vi "manage errors.vi"(8 "error in (no error)":errorcluster, 11 "Channel in":refnum<class "Channel.lvclass">) -> (0 "error out":errorcluster, 1 "sys error":errorcluster, 2 "exe error":errorcluster, 3 "Channel out":refnum<class "Channel.lvclass">)   [LabVIEW 2018, in "Channel.lvclass"]
uses:
  Channel.lvclass
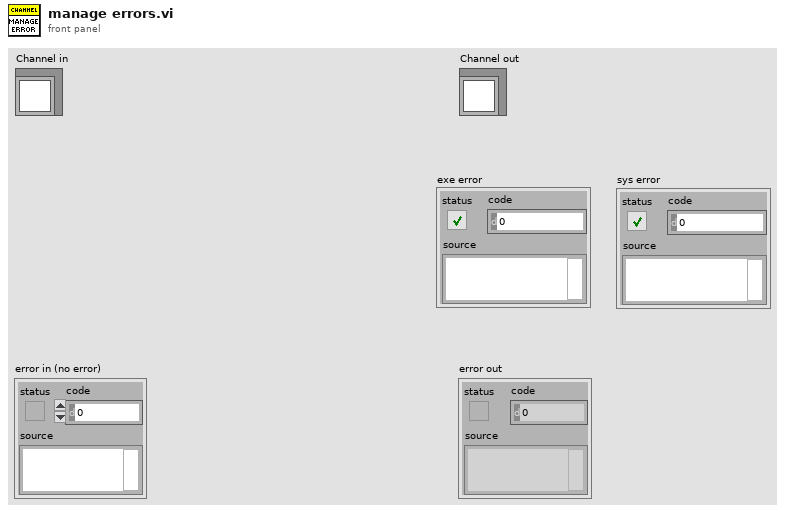
[diagram p1: front panel]
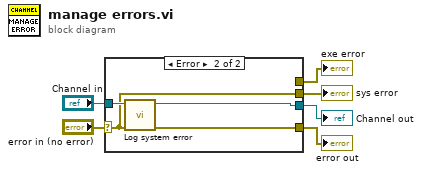
[diagram p0: block diagram]
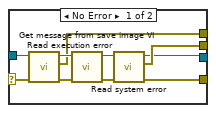
[diagram p2: hidden frame]
diagram:
  n1 = case shown="Error" "error in (no error)" {
    selector: "error in (no error)" -> [w14 w17]
    tunnel: [w7 w20] -> w6
    tunnel: [w8 w19] -> w5
    tunnel: "Channel in" -> [w13 w18]
    tunnel: [w9 w17] -> w4
    tunnel: [w12 _] -> w3
    frame No Error {
      n2 = call-dynamic "Read execution error.vi"("error in (no error)"=w14, "Channel in"=w13) -> ("error out"=w15:errorcluster, "execution error"=w12:errorcluster, "Channel out"=w16:refnum<class "Channel.lvclass">)  [unwired: 7 in]
      n3 = call "Get message from save image VI.vi"("error in (no error)"=w15, "Channel in"=w16) -> ("error out"=w11:errorcluster, "Channel out"=w10:refnum<class "Channel.lvclass">)  [unwired: 8 in]
      n4 = call-dynamic "Read system error.vi"("error in (no error)"=w11, "Channel in"=w10) -> ("error out"=w7:errorcluster, "system error"=w9:errorcluster, "Channel out"=w8:refnum<class "Channel.lvclass">)  [unwired: 7 in]
    }
    frame Error {
      n5 = call "Log system error.vi"("error in (no error)"=w17, "Channel in"=w18) -> ("error out"=w20:errorcluster, "Channel out"=w19:refnum<class "Channel.lvclass">)  [unwired: 8 in]
    }
  }
  "error out" <- w6
  "Channel out" <- w5
  "exe error" <- w3
  "sys error" <- w4
